vi "DCC_test_if_active.vi"(8 "Error In":errorcluster, 10 "Module No":i16, 11 "DLL Path":path) -> (0 "Error Out":errorcluster, 2 "Module No":i16, 3 "DLL Path":path)   [LabVIEW 2017]
doc: "The \"DCC Test if active Function\" returns information whether the DCC module specified by \"Module No.\" is active or not. As a result of a wrong initialisation a module can be deactivated. To find out the reason of deactivating the module please use the \"DCC_Get_Init Function\".\n\nAugust 2018\nFrank Quadt\ninfo@becker-hickl.com"
panel:
  # "(c) 2021 Becker & Hickl GmbH\n     All Rights Reserved."
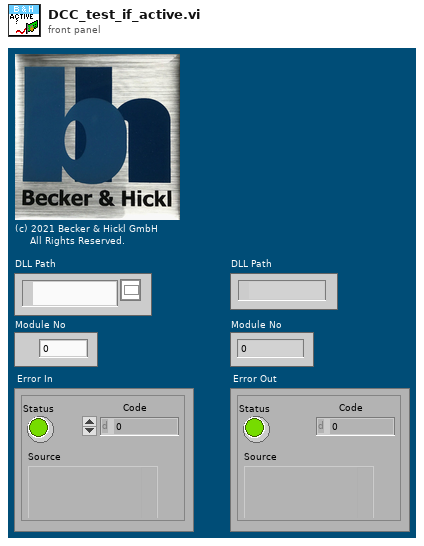
[diagram p1: front panel]
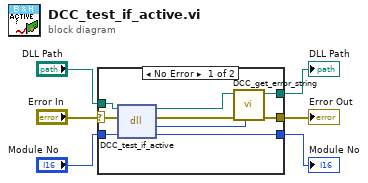
[diagram p0: block diagram]
diagram:
  n1 = case shown="No Error" "Error In" {
    selector: "Error In" -> [w11 w17]
    tunnel: "Module No" -> [w15 w18]
    tunnel: [w14 w18] -> w4
    tunnel: "DLL Path" -> [w12 w16]
    tunnel: [w8 w17] -> w2
    tunnel: [w7 w16] -> w1
    frame No Error {
      n2 = dll-call lib="\\\\bh-fs1\\Archiv/FQ/DCC DLL v.2.4/dcc64.dll" fn="DCC_test_if_active"(path in=w12, error in=w11, "ModuleNo"=w15) -> (path out=w10:path, error out=w9:errorcluster, "return type"=w13:i16, "ModuleNo"=w14:i16)  [unwired: 1 in]
      n3 = call "DCC_get_error_string.vi"("Error ID"=w13, "Error In"=w9, "DLL Path"=w10) -> ("Error Out"=w8:errorcluster, "DLL Path"=w7:path)  [unwired: 6 in, 1 out]
    }
    frame Error {
    }
  }
  "Error Out" <- w2
  "DLL Path" <- w1
  "Module No" <- w4
